vi "CRYSet Front Panel.vi"(8 "Tooltip":string[][](array[string]), 9 "Caption(Boolean Text)":string[][](array[string]), 10 "Control ID and Type(Label Name, Type)":string[][](array[string]), 11 "Vi Ref":refnum<vi>) -> ()   [LabVIEW 2013]
uses:
  CRYMainGlobal.vi
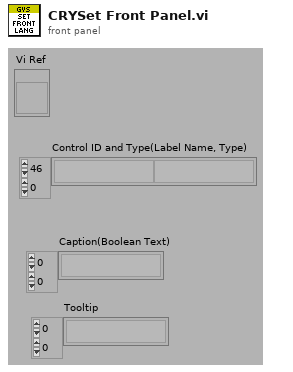
[diagram p1: front panel]
types:
  T1 = enum32{"English", "Chinese", "Korean", "Japanese", "Russian", "Chinese traditional"}
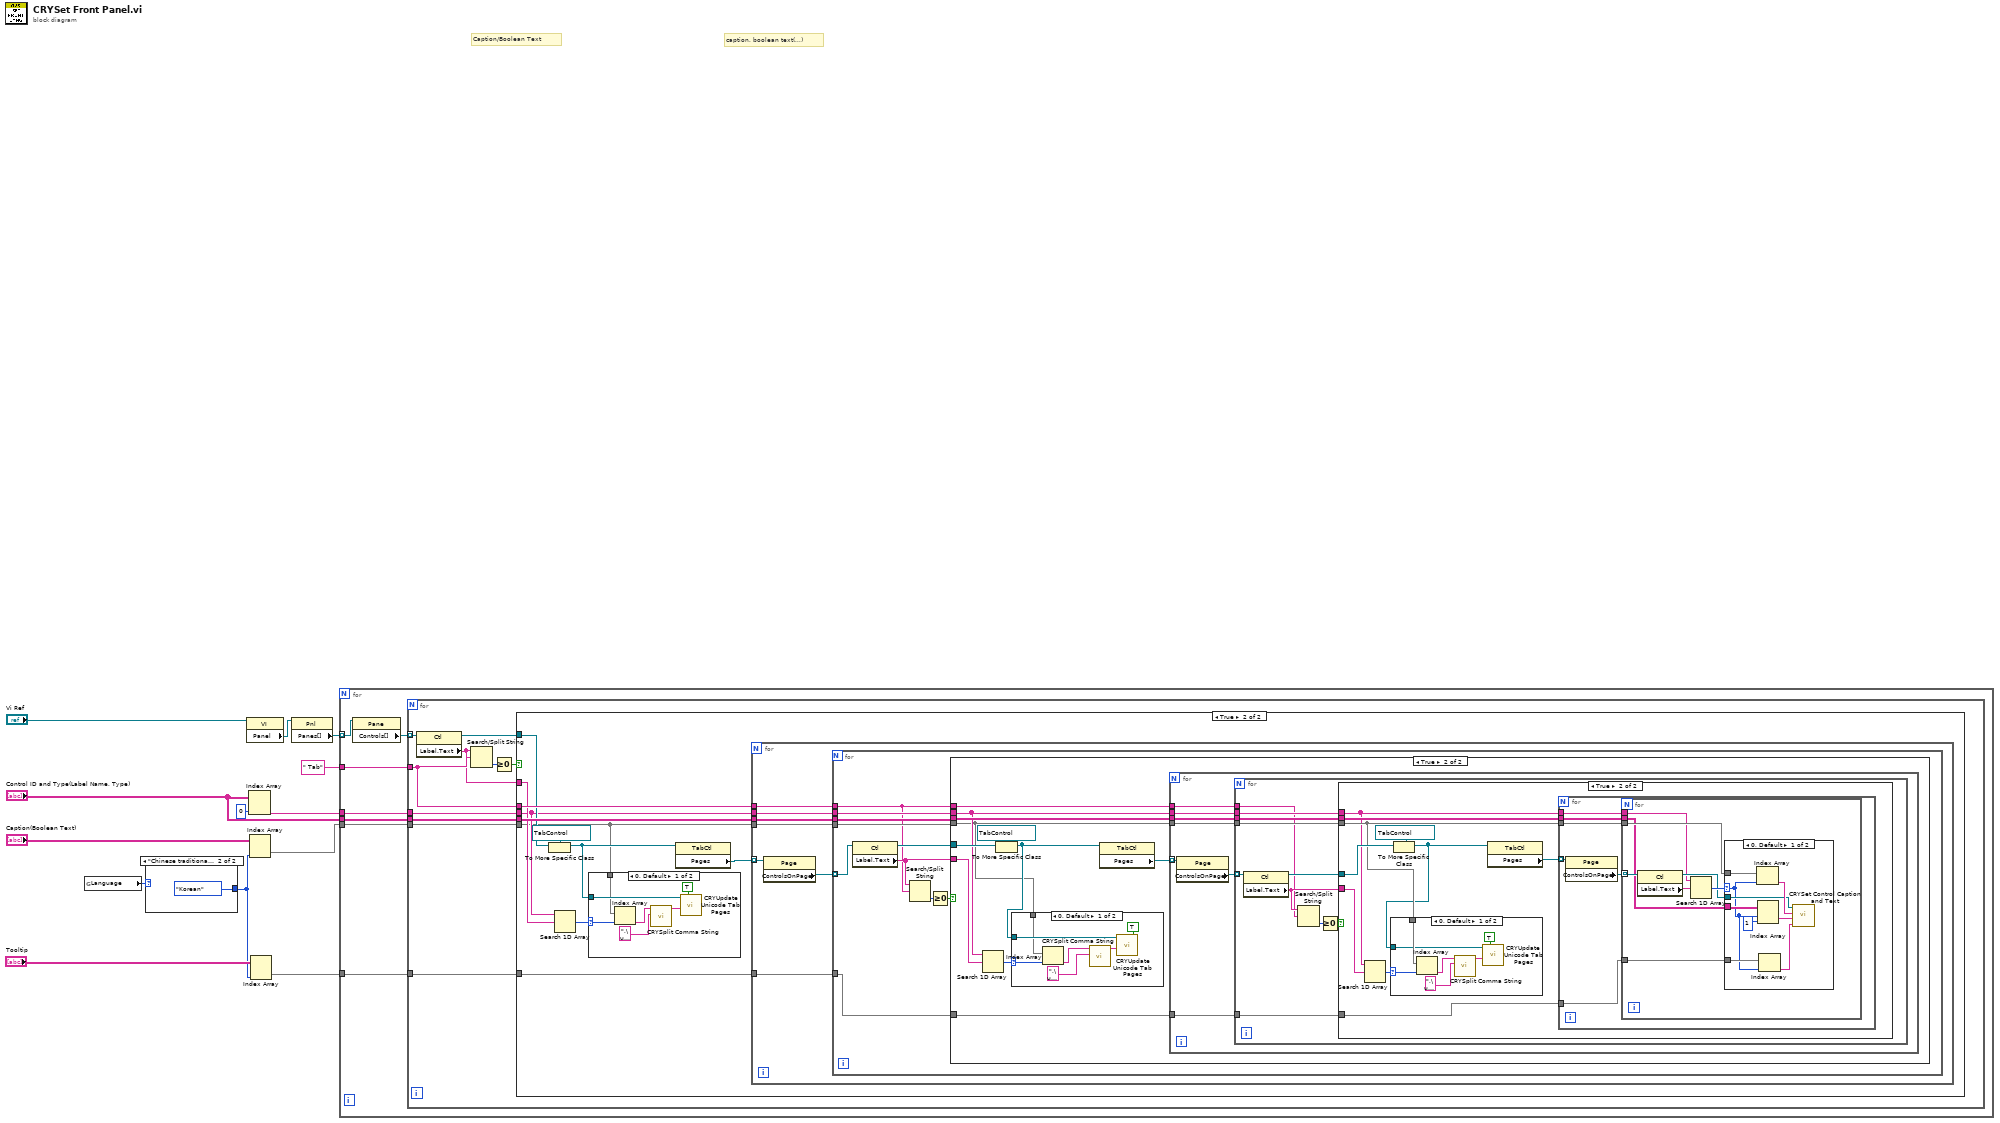
[diagram p0: block diagram]
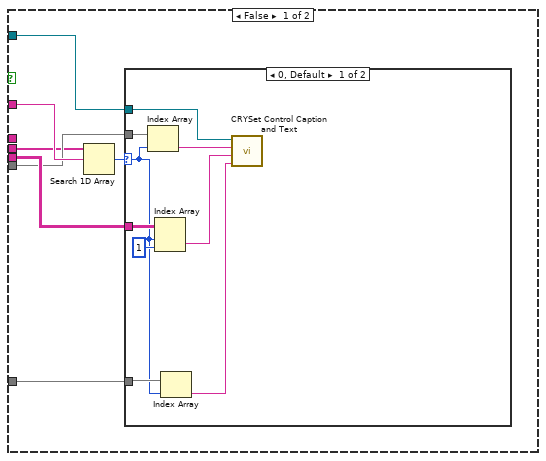
[diagram p3: hidden frame]
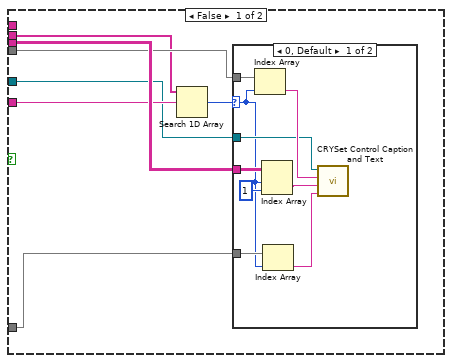
[diagram p6: hidden frame]
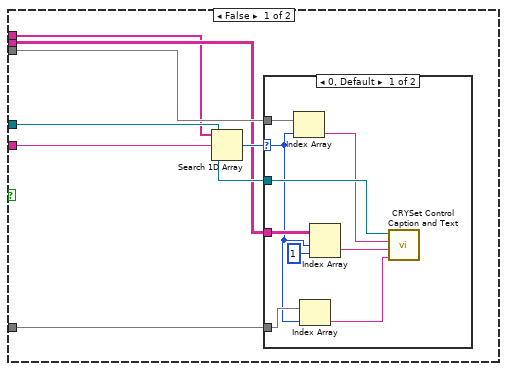
[diagram p9: hidden frame]
diagram:
  # "caption, boolean text(,,,)"
  # "Caption/Boolean Text"
  n1 = global read "CRYMainGlobal.vi" "Language"() -> (w4:T1)
  n2 = case shown="\"Chinese traditional\"" w4 {
    selector: w4 -> [w14 _]
    tunnel: [w14 T1."Korean" ("Language")] -> w2
    frame "English", Default {
    }
    frame "Chinese traditional" {
    }
  }
  n3 = property class="VI"(reference="Vi Ref") -> ("Panel"=w13:refnum<vi>)  [unwired: 1 in, 2 out]
  n4 = Index Array(array="Control ID and Type(Label Name, Type)", index (col)=0 ("index (row)")) -> (element=w9:string[])  [unwired: 1 in]
  n5 = Index Array(array="Caption(Boolean Text)", index (col)=w2) -> (element=w5:string[])  [unwired: 1 in]
  n6 = Index Array(array="Tooltip", index (col)=w2) -> (element=w1:string[])  [unwired: 1 in]
  n7 = property class="Pnl"(reference=w13) -> ("Panes[]"=w12:refnum<vi>[])  [unwired: 1 in, 2 out]
  n8 = for {
    tunnel: w12 -> [w21] mode=indexing
    tunnel: "Control ID and Type(Label Name, Type)" -> [w20]
    tunnel: w5 -> [w19]
    tunnel: w9 -> [w18]
    tunnel: " Tab" ("search string") -> [w17]
    tunnel: w1 -> [w16]
    n9 = property class="Pane"(reference=w21) -> ("Controls[]"=w22:refnum<vi>[])  [unwired: 1 in, 2 out]
    n10 = for {
      tunnel: w22 -> [w32] mode=indexing
      tunnel: w20 -> [w28]
      tunnel: w19 -> [w27]
      tunnel: w18 -> [w26]
      tunnel: w17 -> [w25]
      tunnel: w16 -> [w23]
      n11 = property class="Ctl"(reference=w32) -> (reference out=w29:refnum<vi>, "Label.Text"=w24:string)  [unwired: 1 in, 1 out]
      n12 = Search/Split String(string=w24, search string/char (-)=w25) -> (offset of match=w31:i32)  [unwired: 1 in, 2 out]
      n13 = Greater Or Equal To 0?(x=w31) -> (x >= 0?=w30:bool)
      n14 = case shown="True" w30 {
        tunnel: w29 -> [w35 w55]
        tunnel: w24 -> [w38 w54]
        tunnel: w28 -> [w39 w57]
        tunnel: w27 -> [w36 w50]
        tunnel: w26 -> [w34 w53]
        tunnel: w25 -> [_ w56]
        tunnel: w23 -> [w33 w49]
        frame False {
          n15 = Search 1D Array(1D array=w34, element=w38) -> (index of element=w37:i32)  [unwired: 1 in]
          n16 = case shown="0, Default" w37 {
            selector: w37 -> [w41 _]
            tunnel: w35 -> [w45 _]
            tunnel: w36 -> [w48 _]
            tunnel: w39 -> [w47 _]
            tunnel: w33 -> [w42 _]
            frame 0, Default {
              n17 = Index Array(array=w48, index=w41) -> (element=w44:string)
              n18 = Index Array(array=w47, index (row)=w41, index (col)=1 ("disabled index (col)")) -> (element=w43:string)
              n19 = Index Array(array=w42, index=w41) -> (element=w40:string)
              n20 = call "CRYSet Control Caption and Text.vi"("Tooltip"=w40, "Control Type"=w43, "Caption"=w44, "Control reference In"=w45) -> ()  [unwired: 7 in, 1 out]
            }
            frame -1 {
            }
          }
        }
        frame True {
          n21 = To More Specific Class(target class=refnum<vi> refnum ("Tab Control"), reference=w55) -> (specific class reference=w51:refnum<vi>)  [unwired: 1 in, 1 out]
          n22 = Search 1D Array(1D array=w53, element=w54) -> (index of element=w52:i32)  [unwired: 1 in]
          n23 = case shown="0, Default" w52 {
            selector: w52 -> [w63 _]
            tunnel: w51 -> [w66 _]
            tunnel: w50 -> [w64 _]
            frame 0, Default {
              n24 = Index Array(array=w64, index=w63) -> (element=w62:string)
              n25 = call "CRYSplit Comma String.vi"("sSplit Letter"=",\u0000" ("Label.Text"), "sData Out"=w62) -> ("Array"=w65:string[])  [unwired: 9 in]
              n26 = call "CRYUpdate Unicode Tab Pages.vi"("Interpret as Unicode (T)"=TRUE, "Page Captions"=w65, "Tab Control"=w66) -> ()  [unwired: 5 in, 2 out]
            }
            frame -1 {
            }
          }
          n27 = property class="TabCtl"(reference=w51) -> ("Pages"=w59:refnum<vi>[])  [unwired: 1 in, 2 out]
          n28 = for {
            tunnel: w59 -> [w72] mode=indexing
            tunnel: w50 -> [w71]
            tunnel: w57 -> [w70]
            tunnel: w53 -> [w69]
            tunnel: w56 -> [w68]
            tunnel: w49 -> [w67]
            n29 = property class="Page"(reference=w72) -> ("ControlsOnPage"=w73:refnum<vi>[])  [unwired: 1 in, 2 out]
            n30 = for {
              tunnel: w73 -> [w82] mode=indexing
              tunnel: w71 -> [w79]
              tunnel: w70 -> [w78]
              tunnel: w69 -> [w76]
              tunnel: w68 -> [w75]
              tunnel: w67 -> [w74]
              n31 = property class="Ctl"(reference=w82) -> (reference out=w80:refnum<vi>, "Label.Text"=w77:string)  [unwired: 1 in, 1 out]
              n32 = Search/Split String(string=w77, search string/char (-)=w75) -> (offset of match=w83:i32)  [unwired: 1 in, 2 out]
              n33 = Greater Or Equal To 0?(x=w83) -> (x >= 0?=w81:bool)
              n34 = case shown="True" w81 {
                tunnel: w80 -> [w86 w110]
                tunnel: w79 -> [w88 w101]
                tunnel: w78 -> [w89 w107]
                tunnel: w77 -> [w87 w103]
                tunnel: w76 -> [w85 w105]
                tunnel: w75 -> [_ w104]
                tunnel: w74 -> [w84 w100]
                frame False {
                  n35 = Search 1D Array(1D array=w85, element=w87) -> (index of element=w90:i32)  [unwired: 1 in]
                  n36 = case shown="0, Default" w90 {
                    selector: w90 -> [w92 _]
                    tunnel: w86 -> [w94 _]
                    tunnel: w88 -> [w99 _]
                    tunnel: w89 -> [w98 _]
                    tunnel: w84 -> [w93 _]
                    frame 0, Default {
                      n37 = Index Array(array=w99, index=w92) -> (element=w95:string)
                      n38 = Index Array(array=w98, index (row)=w92, index (col)=1 ("disabled index (col)")) -> (element=w96:string)
                      n39 = Index Array(array=w93, index=w92) -> (element=w91:string)
                      n40 = call "CRYSet Control Caption and Text.vi"("Tooltip"=w91, "Control Type"=w96, "Caption"=w95, "Control reference In"=w94) -> ()  [unwired: 7 in, 1 out]
                    }
                    frame -1 {
                    }
                  }
                }
                frame True {
                  n41 = Search 1D Array(1D array=w105, element=w103) -> (index of element=w106:i32)  [unwired: 1 in]
                  n42 = To More Specific Class(target class=refnum<vi> refnum ("Tab Control"), reference=w110) -> (specific class reference=w102:refnum<vi>)  [unwired: 1 in, 1 out]
                  n43 = case shown="0, Default" w106 {
                    selector: w106 -> [w114 _]
                    tunnel: w102 -> [w117 _]
                    tunnel: w101 -> [w115 _]
                    frame 0, Default {
                      n44 = Index Array(array=w115, index=w114) -> (element=w113:string)
                      n45 = call "CRYSplit Comma String.vi"("sSplit Letter"=",\u0000" ("Label.Text"), "sData Out"=w113) -> ("Array"=w116:string[])  [unwired: 9 in]
                      n46 = call "CRYUpdate Unicode Tab Pages.vi"("Interpret as Unicode (T)"=TRUE, "Page Captions"=w116, "Tab Control"=w117) -> ()  [unwired: 5 in, 2 out]
                    }
                    frame -1 {
                    }
                  }
                  n47 = property class="TabCtl"(reference=w102) -> ("Pages"=w109:refnum<vi>[])  [unwired: 1 in, 2 out]
                  n48 = for {
                    tunnel: w109 -> [w124] mode=indexing
                    tunnel: w101 -> [w122]
                    tunnel: w107 -> [w121]
                    tunnel: w105 -> [w120]
                    tunnel: w104 -> [w119]
                    tunnel: w100 -> [w118]
                    n49 = property class="Page"(reference=w124) -> ("ControlsOnPage"=w123:refnum<vi>[])  [unwired: 1 in, 2 out]
                    n50 = for {
                      tunnel: w123 -> [w132] mode=indexing
                      tunnel: w122 -> [w134]
                      tunnel: w121 -> [w133]
                      tunnel: w120 -> [w127]
                      tunnel: w119 -> [w126]
                      tunnel: w118 -> [w125]
                      n51 = property class="Ctl"(reference=w132) -> (reference out=w131:refnum<vi>, "Label.Text"=w129:string)  [unwired: 1 in, 1 out]
                      n52 = Search/Split String(string=w129, search string/char (-)=w126) -> (offset of match=w130:i32)  [unwired: 1 in, 2 out]
                      n53 = Greater Or Equal To 0?(x=w130) -> (x >= 0?=w128:bool)
                      n54 = case shown="True" w128 {
                        tunnel: w134 -> [w140 w155]
                        tunnel: w133 -> [w137 w160]
                        tunnel: w131 -> [w139 w158]
                        tunnel: w129 -> [w138 w152]
                        tunnel: w127 -> [w136 w153]
                        tunnel: w125 -> [w135 w151]
                        frame False {
                          n55 = Search 1D Array(1D array=w136, element=w138) -> (index of element=w141:i32)  [unwired: 1 in]
                          n56 = case shown="0, Default" w141 {
                            selector: w141 -> [w143 _]
                            tunnel: w139 -> [w147 _]
                            tunnel: w140 -> [w150 _]
                            tunnel: w137 -> [w148 _]
                            tunnel: w135 -> [w144 _]
                            frame 0, Default {
                              n57 = Index Array(array=w150, index=w143) -> (element=w146:string)
                              n58 = Index Array(array=w144, index=w143) -> (element=w142:string)
                              n59 = Index Array(array=w148, index (row)=w143, index (col)=1 ("disabled index (col)")) -> (element=w145:string)
                              n60 = call "CRYSet Control Caption and Text.vi"("Tooltip"=w142, "Control Type"=w145, "Caption"=w146, "Control reference In"=w147) -> ()  [unwired: 7 in, 1 out]
                            }
                            frame -1 {
                            }
                          }
                        }
                        frame True {
                          n61 = Search 1D Array(1D array=w153, element=w152) -> (index of element=w156:i32)  [unwired: 1 in]
                          n62 = To More Specific Class(target class=refnum<vi> refnum ("Tab Control"), reference=w158) -> (specific class reference=w154:refnum<vi>)  [unwired: 1 in, 1 out]
                          n63 = case shown="0, Default" w156 {
                            selector: w156 -> [w165 _]
                            tunnel: w154 -> [w162 _]
                            tunnel: w155 -> [w166 _]
                            frame 0, Default {
                              n64 = Index Array(array=w166, index=w165) -> (element=w164:string)
                              n65 = call "CRYSplit Comma String.vi"("sSplit Letter"=",\u0000" ("Label.Text"), "sData Out"=w164) -> ("Array"=w167:string[])  [unwired: 9 in]
                              n66 = call "CRYUpdate Unicode Tab Pages.vi"("Interpret as Unicode (T)"=TRUE, "Page Captions"=w167, "Tab Control"=w162) -> ()  [unwired: 5 in, 2 out]
                            }
                            frame -1 {
                            }
                          }
                          n67 = property class="TabCtl"(reference=w154) -> ("Pages"=w157:refnum<vi>[])  [unwired: 1 in, 2 out]
                          n68 = for {
                            tunnel: w155 -> [w173]
                            tunnel: w160 -> [w172]
                            tunnel: w157 -> [w171] mode=indexing
                            tunnel: w153 -> [w169]
                            tunnel: w151 -> [w168]
                            n69 = property class="Page"(reference=w171) -> ("ControlsOnPage"=w170:refnum<vi>[])  [unwired: 1 in, 2 out]
                            n70 = for {
                              tunnel: w173 -> [w180]
                              tunnel: w172 -> [w176]
                              tunnel: w170 -> [w179] mode=indexing
                              tunnel: w169 -> [w175]
                              tunnel: w168 -> [w174]
                              n71 = property class="Ctl"(reference=w179) -> (reference out=w177:refnum<vi>, "Label.Text"=w178:string)  [unwired: 1 in, 1 out]
                              n72 = Search 1D Array(1D array=w175, element=w178) -> (index of element=w181:i32)  [unwired: 1 in]
                              n73 = case shown="0, Default" w181 {
                                selector: w181 -> [w184 _]
                                tunnel: w177 -> [w186 _]
                                tunnel: w180 -> [w190 _]
                                tunnel: w176 -> [w189 _]
                                tunnel: w174 -> [w185 _]
                                frame 0, Default {
                                n74 = Index Array(array=w190, index=w184) -> (element=w187:string)
                                n75 = Index Array(array=w189, index (row)=w184, index (col)=1 ("disabled index (col)")) -> (element=w183:string)
                                n76 = Index Array(array=w185, index=w184) -> (element=w182:string)
                                n77 = call "CRYSet Control Caption and Text.vi"("Tooltip"=w182, "Control Type"=w183, "Caption"=w187, "Control reference In"=w186) -> ()  [unwired: 7 in, 1 out]
                                }
                                frame -1 {
                                }
                              }
                            }
                          }
                        }
                      }
                    }
                  }
                }
              }
            }
          }
        }
      }
    }
  }
